vi "Deliver Cube.vi"(9 "run?":dbl, 10 "Angle":dbl, 11 "Scale?":bool) -> (1 "out":dbl)   [LabVIEW 2017]
uses:
  Robot Global Data.vi
  <vilib>/Rock Robotics/WPI/Utilities/WPI_GetSetVariantRefNum.vi
  <vilib>/Rock Robotics/WPI/ThirdParty/Phoenix-LabVIEW/Motor Controller/Get/CTRE_Phoenix_MotorController_GetQuadratureData.vi
  <vilib>/Rock Robotics/WPI/RobotDrive/WPI_RobotDriveArcadeDrive_Standard(NoSaturation).vi
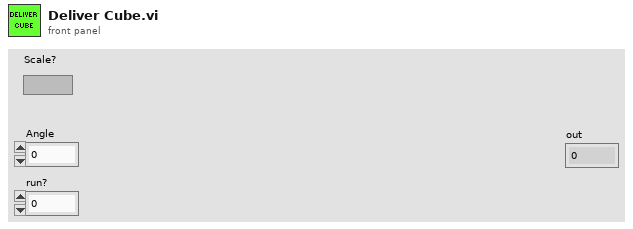
[diagram p1: front panel]
types:
  T1 = typedef "WPI_RobotDriveDevRef.ctl" = cluster{"DevStatus":errorcluster, "Motors[]":T2[], "Square Inputs":bool, "Max Output":dbl}
  T2 = typedef "WPI_MotorControlDeviceRef.ctl" = cluster{"DeviceStatus":errorcluster, "Type":T3, "PWM":cluster{"PWM Channel":T4, "DeadBand":T5}, "CAN":cluster{"Device Number":u8, "SetOutput VI Ref":variant, "GetOutput VI Ref":variant, "Enable VI Ref":variant, "Disable VI Ref":variant, "Data":variant}, "Invert":bool, "DIO PWM":cluster{"PWM \"Enable\" Channel":T4, "DIOChannel":T6, "PWM Rate":dbl}}
  T3 = typedef "WPI_MotorControlType.ctl" = enum16{"PWM", "CAN", "DIO PWM"}
  T4 = typedef "FPGA_DIOPWMChannel.ctl" = enum8{"PWM 0", "PWM 1", "PWM 2", "PWM 3", "PWM 4", "PWM 5", "PWM 6", "PWM 7", "PWM 8", "PWM 9", "PWM MXP 0", "PWM MXP 1", "PWM MXP 2", "PWM MXP 3", "PWM MXP 4", "PWM MXP 5", "PWM MXP 6", "PWM MXP 7", "PWM MXP 8", "PWM MXP 9", "Invalid"}
  T5 = typedef "WPI_PWMDeadband.ctl" = cluster{"Name":string, "maxPositivePwm":i32, "minPositivePwm":i32, "centerPwm":i32, "maxNegativePwm":i32, "minNegativePwm":i32, "angularRange":u16}
  T6 = typedef "FPGA_DIOChannel.ctl" = enum8{"DIO 0", "DIO 1", "DIO 2", "DIO 3", "DIO 4", "DIO 5", "DIO 6", "DIO 7", "DIO 8", "DIO 9", "DIO MXP 0", "DIO MXP 1", "DIO MXP 2", "DIO MXP 3", "DIO MXP 4", "DIO MXP 5", "DIO MXP 6", "DIO MXP 7", "DIO MXP 8", "DIO MXP 9", "DIO MXP 10", "DIO MXP 11", "DIO MXP 12", "DIO MXP 13", "DIO MXP 14", "DIO MXP 15", "SPI Port CS1", "SPI Port CS2", "SPI Port CS3", "SPI Port MISO", "SPI Port MOSI", "Invalid"}
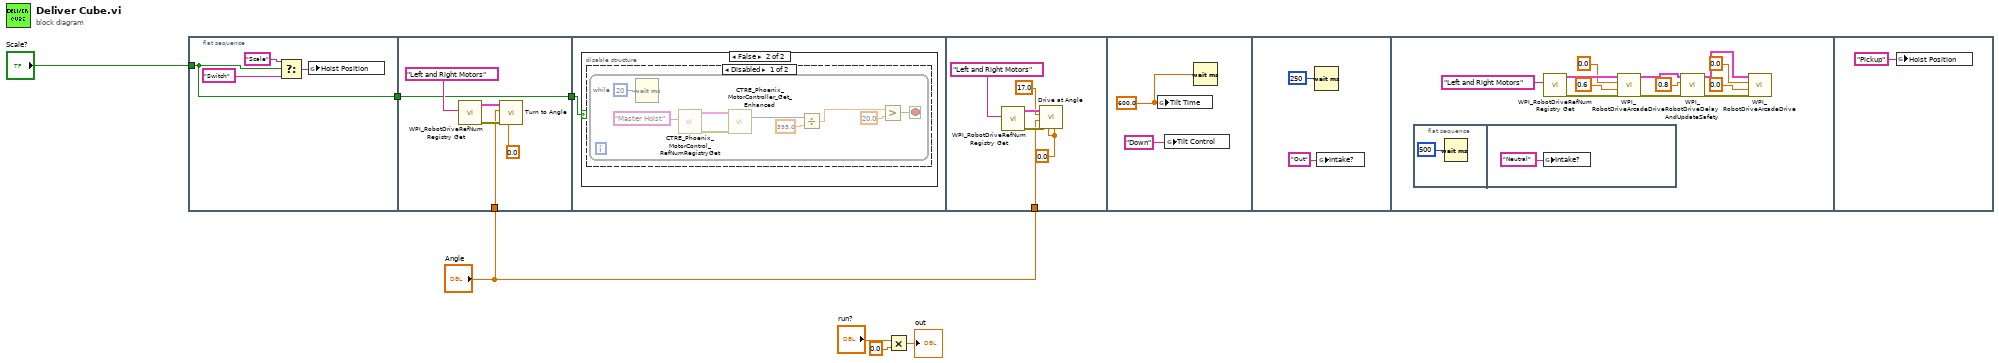
[diagram p0: block diagram]
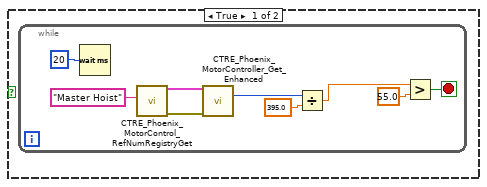
[diagram p2: hidden frame]
diagram:
  n1 = flat-sequence {
    tunnel: "Scale?" -> [w8]
    tunnel: [w8] -> w2
    tunnel: "Angle" -> [w14]
    tunnel: w2 -> [w12]
    tunnel: [w12] -> w1
    tunnel: w1 -> [w18]
    tunnel: "Angle" -> [w38]
    frame #0 {
      n2 = Select(t="Scale", s=w8, f="Switch") -> (s? t:f=w11:string)
      n3 = global write "Robot Global Data.vi" "Hoist Position"(w11) -> ()
    }
    frame #1 {
      n4 = call <vilib>:"WPI_RobotDriveRefNum Registry Get.vi"("refnum name"="Left and Right Motors") -> ("error out"=w17:errorcluster, "RobotDriveDevRef"=w16:T1)  [unwired: 9 in]
      n5 = call "Turn to Angle.vi"("in power"=0.0, "error in (no error)"=w17, "Angle"=w14, "RobotDriveDevRef"=w16) -> ()  [unwired: 5 in, 3 out]
    }
    frame #2 {
      n6 = case shown="False" w18 {
        frame True {
          n7 = while {
            stop <- w21 stop-if-true
            n8 = Wait (ms)(milliseconds to wait=u32 20) -> ()  [unwired: 1 out]
            n9 = call <vilib>:"CTRE_Phoenix_MotorControl_RefNumRegistryGet.vi"("refnum name"="Master Hoist") -> ("error out"=w27:errorcluster, "PhoenixMotorControlDevRef"=w26:T2)  [unwired: 9 in]
            n10 = call-poly <vilib>:"CTRE_Phoenix_MotorController_Get_Enhanced.vi"("PhoenixMotorControlDevRef"=w26, "error in"=w27) -> ("Quadrature Position"=w19:i32)  [unwired: 10 in, 3 out]
            n11 = Divide(x=w19, y=395.0) -> (x/y=w22:dbl)
            n12 = Greater?(x=w22, y=55.0) -> (0:w21:bool)
          }
        }
        frame False {
          n13 = disable-structure shown="Disabled" {
            frame Disabled {
              n14 = while {
                stop <- w30 stop-if-true
                n15 = Wait (ms)(milliseconds to wait=u32 20) -> ()  [unwired: 1 out]
                n16 = call <vilib>:"CTRE_Phoenix_MotorControl_RefNumRegistryGet.vi"("refnum name"="Master Hoist") -> ("error out"=w36:errorcluster, "PhoenixMotorControlDevRef"=w35:T2)  [unwired: 9 in]
                n17 = call-poly <vilib>:"CTRE_Phoenix_MotorController_Get_Enhanced.vi"("PhoenixMotorControlDevRef"=w35, "error in"=w36) -> ("Quadrature Position"=w28:i32)  [unwired: 10 in, 3 out]
                n18 = Divide(x=w28, y=395.0) -> (x/y=w31:dbl)
                n19 = Greater?(x=w31, y=20.0) -> (0:w30:bool)
              }
            }
            frame Enabled {
            }
          }
        }
      }
    }
    frame #3 {
      w37 = 0.0
      n20 = call <vilib>:"WPI_RobotDriveRefNum Registry Get.vi"("refnum name"="Left and Right Motors") -> ("error out"=w42:errorcluster, "RobotDriveDevRef"=w41:T1)  [unwired: 9 in]
      n21 = call "Drive at Angle.vi"("end power"=w37, "Begin power"=w37, "error in (no error)"=w42, "Angle"=w38, "Distance"=17.0, "RobotDriveDevRef"=w41) -> ()  [unwired: 3 in, 3 out]
    }
    frame #4 {
      w43 = 600.0 ("Tilt Time")
      n22 = global write "Robot Global Data.vi" "Tilt Time"(w43) -> ()
      n23 = global write "Robot Global Data.vi" "Tilt Control"("Down" ("Tilt Control")) -> ()
      n24 = Wait (ms)(milliseconds to wait=w43) -> ()  [unwired: 1 out]
    }
    frame #5 {
      n25 = Wait (ms)(milliseconds to wait=u32 250) -> ()  [unwired: 1 out]
      n26 = global write "Robot Global Data.vi" "Intake?"("Out" ("Intake?")) -> ()
    }
    frame #6 {
      n27 = flat-sequence {
        frame #0 {
          n28 = Wait (ms)(milliseconds to wait=u32 500) -> ()  [unwired: 1 out]
        }
        frame #1 {
          n29 = global write "Robot Global Data.vi" "Intake?"("Neutral" ("Intake?")) -> ()
        }
      }
      n30 = call <vilib>:"WPI_RobotDriveRefNum Registry Get.vi"("refnum name"="Left and Right Motors") -> ("error out"=w53:errorcluster, "RobotDriveDevRef"=w54:T1)  [unwired: 9 in]
      n31 = call-poly <vilib>:"WPI_RobotDriveArcadeDrive.vi"("error in (no error)"=w53, "Y axis value"=0.6, "X axis value"=0.0, "RobotDriveDevRef"=w54) -> ("error out"=w55:errorcluster, "RobotDriveDevRef"=w56:T1)  [unwired: 5 in, 1 out]
      n32 = call <vilib>:"WPI_RobotDriveDelayAndUpdateSafety.vi"("error in (no error)"=w55, "Delay (s)"=0.8, "RobotDriveDevRef"=w56) -> ("error out"=w57:errorcluster, "RobotDriveDevRef 2"=w58:T1)  [unwired: 7 in]
      n33 = call-poly <vilib>:"WPI_RobotDriveArcadeDrive.vi"("error in (no error)"=w57, "Y axis value"=0.0, "X axis value"=0.0, "RobotDriveDevRef"=w58) -> ()  [unwired: 5 in, 3 out]
    }
    frame #7 {
      n34 = global write "Robot Global Data.vi" "Hoist Position"("Pickup" ("Hoist Position")) -> ()
    }
  }
  n35 = Multiply(x="run?", y=0.0) -> (x*y=→"out":dbl)
